vi "Anritsu VNA Trigger and Fetch Measurement.vi"(6 "Channel":i8=1 min=1 step=1, 7 "Anritsu VNA":T1, 8 "error in (no error)":errorcluster, 9 "Timeout, ms (10000)":u32=10000, 11 "VISA Resource Name":refnum<visa-resource-name>) -> (0 "error out":errorcluster, 3 "dup VISA Resource Name":refnum<visa-resource-name>)   [LabVIEW 2011]
doc: "Takes a SING sweep and returns the magnitude in dB of the requested data"
uses:
  TypeDefs/Anritsu VNA Instrument Info.ctl
  TypeDefs/Anritsu VNA Trigger Mode.ctl
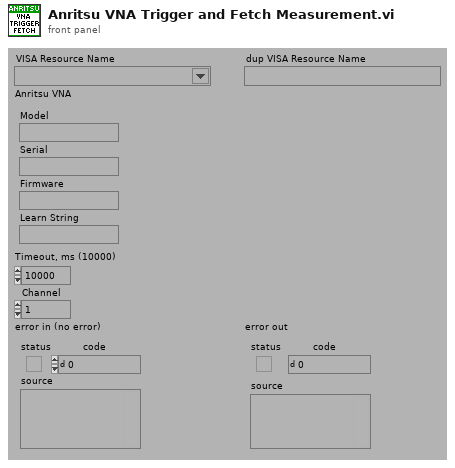
[diagram p1: front panel]
types:
  T1 = typedef "Anritsu VNA Instrument Info.ctl" = cluster{"Model":string, "Serial":string, "Firmware":string, "Learn String":string}
  T2 = typedef "Anritsu VNA Model.ctl" = enum16{"Not Supported", "37XXXX", "MS20XXX", "MS462XX", "MS464XX"}
  T3 = typedef "Anritsu VNA Trigger Mode.ctl" = enum16{"Continuous", "Hold", "Single"}
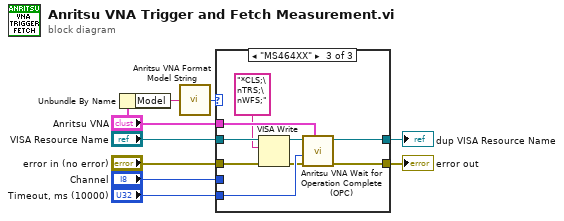
[diagram p0: block diagram]
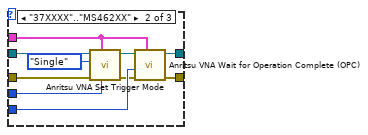
[diagram p3: hidden frame]
diagram:
  n1 = Unbundle By Name("Anritsu VNA") -> ("Model"=w2:string)
  n2 = call "Anritsu VNA Format Model String.vi"("Model"=w2) -> ("Model"=w1:T2)
  n3 = case shown="\"MS464XX\"" w1 {
    tunnel: [w10 w21 w30] -> w9
    tunnel: [w11 w20 w29] -> w8
    tunnel: "Timeout, ms (10000)" -> [_ w19 w28]
    tunnel: "Anritsu VNA" -> [_ w16 w27]
    tunnel: "error in (no error)" -> [w10 w15 w26]
    tunnel: "VISA Resource Name" -> [w11 w13 w23]
    tunnel: "Channel" -> [_ w12 _]
    frame "Not Supported" {
    }
    frame "37XXXX".."MS462XX" {
      n4 = call "Anritsu VNA Set Trigger Mode.vi"("Channel"=w12, "Anritsu VNA"=w16, "error in (no error)"=w15, "Trigger Mode"=Anritsu_VNA_Trigger_Mode."Single", "VISA Resource Name"=w13) -> ("error out"=w18:errorcluster, "dup VISA Resource Name"=w17:refnum<visa-resource-name>)  [unwired: 5 out]
      n5 = call "Anritsu VNA Wait for Operation Complete (OPC).vi"("Anritsu VNA"=w16, "error in (no error)"=w18, "Timeout, ms (10000)"=w19, "VISA Resource Name"=w17) -> ("error out"=w21:errorcluster, "dup VISA Resource Name"=w20:refnum<visa-resource-name>)  [unwired: 6 out]
    }
    frame "MS464XX" {
      n6 = VISA Write(VISA resource name=w23, write buffer="*CLS;\nTRS;\nWFS;", error in (no error)=w26) -> (VISA resource name out=w24:refnum<visa-resource-name>, error out=w25:errorcluster)  [unwired: 1 out]
      n7 = call "Anritsu VNA Wait for Operation Complete (OPC).vi"("Anritsu VNA"=w27, "error in (no error)"=w25, "Timeout, ms (10000)"=w28, "VISA Resource Name"=w24) -> ("error out"=w30:errorcluster, "dup VISA Resource Name"=w29:refnum<visa-resource-name>)  [unwired: 6 out]
    }
  }
  "dup VISA Resource Name" <- w8
  "error out" <- w9
